vi "Combine Status Monitor and Transient Capture (Multiple UUTs).vi"() -> ()   [LabVIEW 2017]
uses:
  Status Monitor/Status Monitor (Single Unit).vi
  Status Monitor/Status Monitor Library.lvlib
panel:
  out "UUT Name":string
  in  "Soft Trigger":bool
  in  "Post-Trigger Samples":i32=100000
  in  "configuration file path":path
  in  "stop":bool
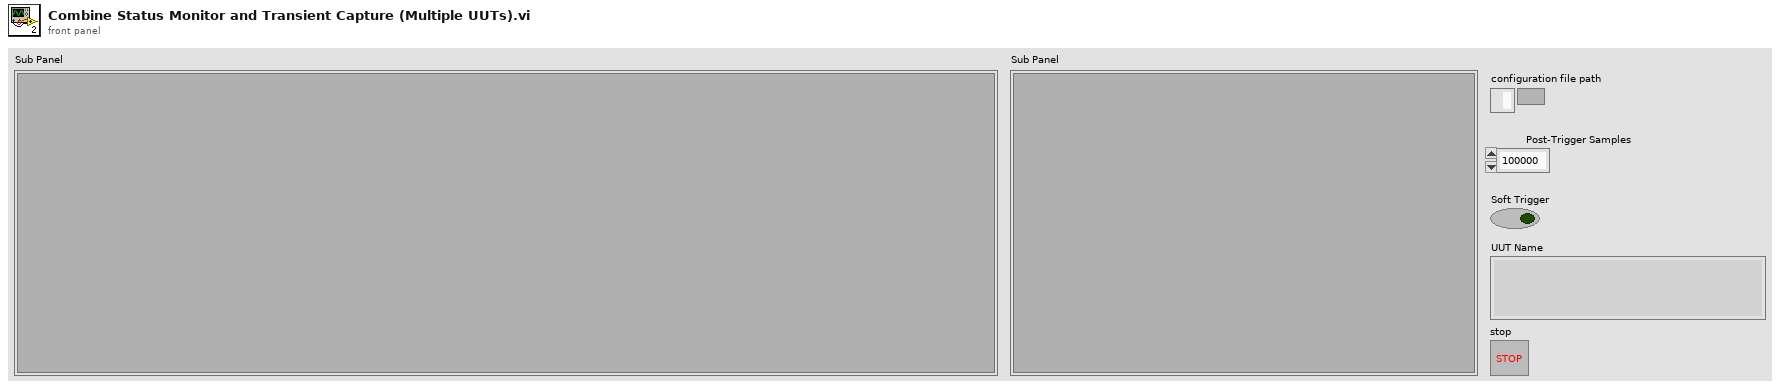
[diagram p1: front panel]
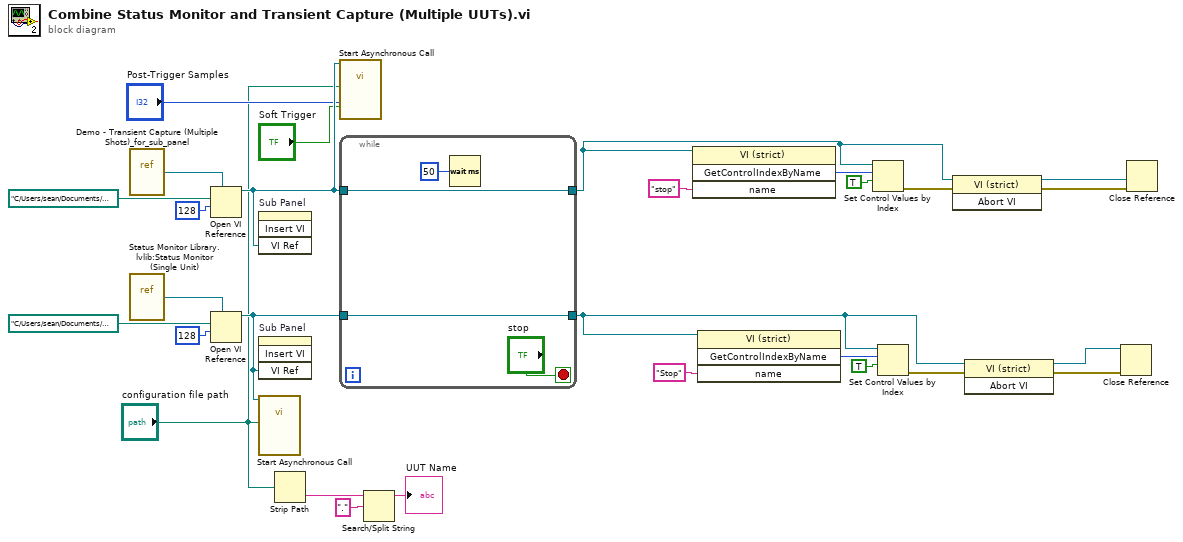
[diagram p0: block diagram]
diagram:
  n1 = vi-ref "Demo - Transient Capture (Multiple Shots)_for_sub_panel.vi"() -> (w26:refnum<vi>)
  n2 = vi-ref "Status Monitor Library.lvlib:Status Monitor (Single Unit).vi"() -> (w23:refnum<vi>)
  n3 = Open VI Reference(type specifier VI Refnum (for type only)=w26, vi path=path "C:/Users/sean/Documents/Workspace/LabVIEW/Sean/acq400_lv/Source Code/Transient Capture (Advanced Demo)/Demo - Transient Capture (Multiple Shots)_for_sub_panel.vi", options=128) -> (vi reference=w27:refnum<vi>)  [unwired: 3 in, 1 out]
  n4 = Open VI Reference(type specifier VI Refnum (for type only)=w23, vi path=path "C:/Users/sean/Documents/Workspace/LabVIEW/Sean/acq400_lv/Source Code/Status Monitor/Status Monitor (Single Unit).vi", options=128) -> (vi reference=w22:refnum<vi>)  [unwired: 3 in, 1 out]
  n5 = invoke on="Sub Panel" class="SubPnl" method="Insert VI"("VI Ref"=w27) -> ()  [unwired: 3 in, 4 out]
  n6 = invoke on="Sub Panel" class="SubPnl" method="Insert VI"("VI Ref"=w22) -> ()  [unwired: 3 in, 4 out]
  n7 = call-by-ref "Start Asynchronous Call"(reference=w22, "configuration file path"="configuration file path") -> ()  [unwired: 12 in, 2 out]
  n8 = Strip Path(path="configuration file path") -> (name=w16:string)  [unwired: 1 out]
  n9 = call-by-ref "Start Asynchronous Call"(reference=w27, "Soft Trigger"="Soft Trigger", "Post-Trigger Samples"="Post-Trigger Samples", "configuration file path"="configuration file path") -> ()  [unwired: 10 in, 2 out]
  n10 = while {
    tunnel: w22 -> [w32]
    tunnel: w27 -> [w31]
    tunnel: [w32] -> w4
    tunnel: [w31] -> w7
    stop <- "stop" stop-if-true
    n11 = Wait (ms)(milliseconds to wait=u32 50) -> ()  [unwired: 1 out]
  }
  n12 = Search/Split String(string=w16, search string/char (-)=".") -> (substring before match=→"UUT Name":string)  [unwired: 1 in, 2 out]
  n13 = invoke class="VI (strict)" method="GetControlIndexByName"(reference=w7, "name"="stop") -> ("GetControlIndexByName"=w13:i32)  [unwired: 2 in, 3 out]
  n14 = invoke class="VI (strict)" method="GetControlIndexByName"(reference=w4, "name"="Stop") -> ("GetControlIndexByName"=w10:i32)  [unwired: 2 in, 3 out]
  n15 = Set Control Values by Index(0:w7, 1:w13, 2:TRUE) -> (11:w5:errorcluster)  [unwired: 1 in]
  n16 = Set Control Values by Index(0:w4, 1:w10, 2:TRUE) -> (11:w3:errorcluster)  [unwired: 1 in]
  n17 = invoke class="VI (strict)" method="Abort VI"(reference=w7, error in=w5) -> (reference out=w8:refnum<vi>, error out=w6:errorcluster)  [unwired: 1 in, 1 out]
  n18 = invoke class="VI (strict)" method="Abort VI"(reference=w4, error in=w3) -> (reference out=w1:refnum<vi>, error out=w2:errorcluster)  [unwired: 1 in, 1 out]
  n19 = Close Reference(reference=w1, error in (no error)=w2) -> ()  [unwired: 1 out]
  n20 = Close Reference(reference=w8, error in (no error)=w6) -> ()  [unwired: 1 out]
